vi "WriteGoodmanInfo.vi"(4 "System Pos Info":T2, 5 "error in (no error)":errorcluster, 6 "# of Entries (before)":i16, 7 "Component Names":T1, 8 "Path to FITS Header File":path) -> (0 "error out":errorcluster, 2 "# of Entries (after)":i16, 3 "Path to FITS Header File":path)   [LabVIEW 2015]
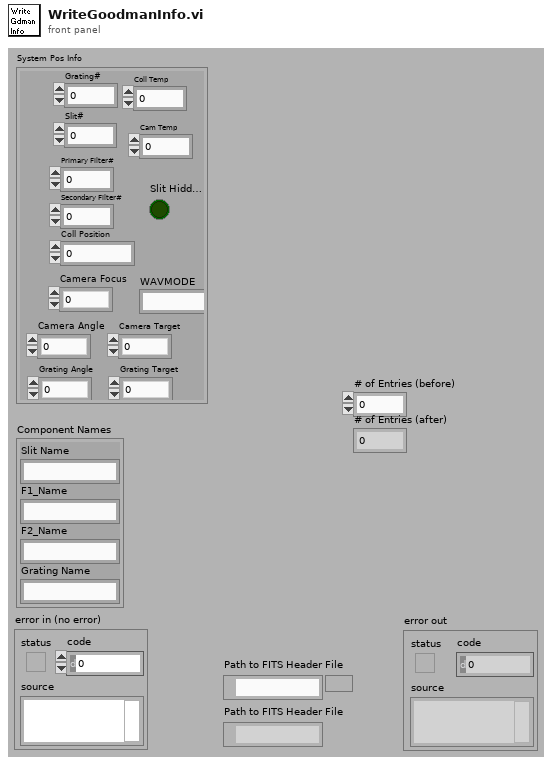
[diagram p1: front panel]
types:
  T1 = cluster{"Slit Name":string, "F1_Name":string, "F2_Name":string, "Grating Name":string}
  T2 = cluster{"Grating#":i32, "Slit#":i32, "Primary Filter#":i32, "Secondary Filter#":i32, "Coll Position":i32, "Camera Focus":i32, "Camera Angle":dbl, "Grating Angle":dbl, "Coll Temp":dbl, "Cam Temp":dbl, "Camera Target":dbl, "Grating Target":dbl, "WAVMODE":string, "Slit Hidden?":bool}
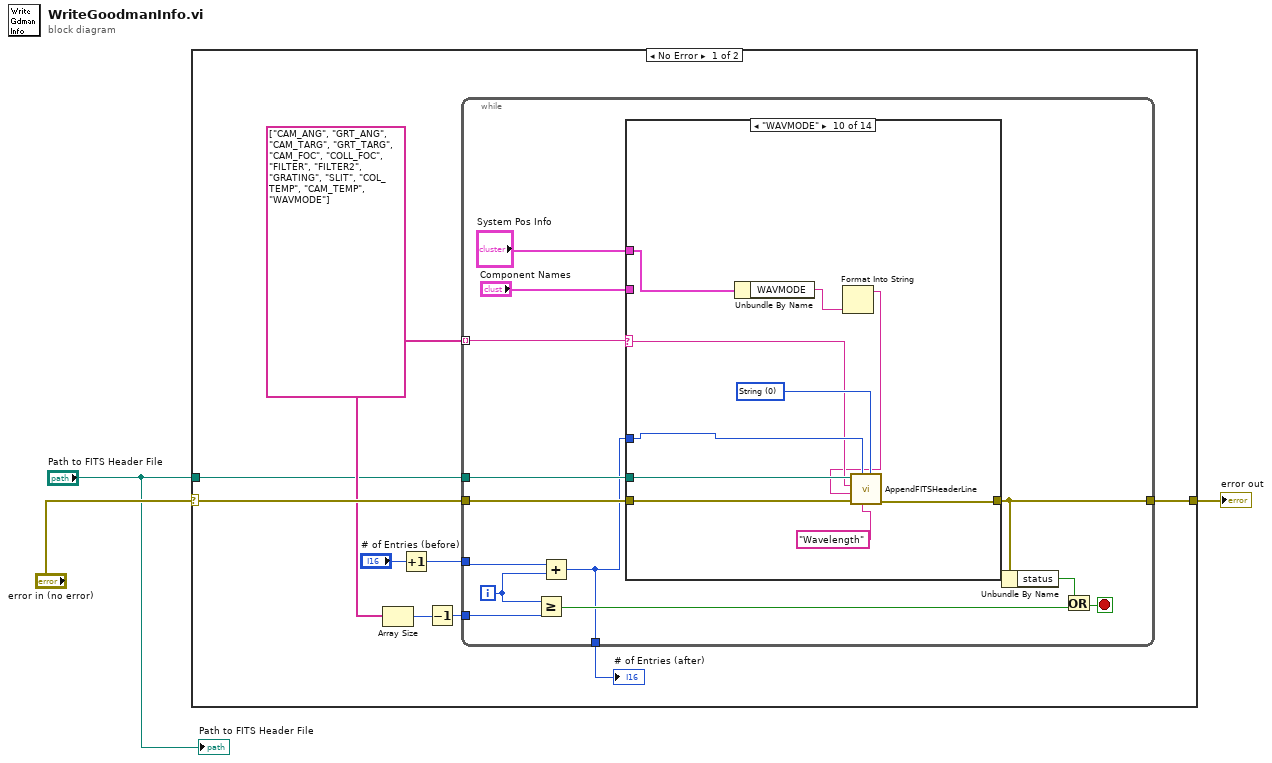
[diagram p0: block diagram]
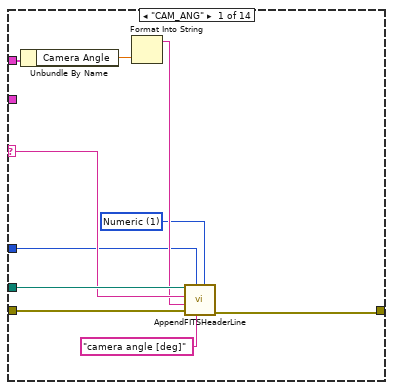
[diagram p2: hidden frame]
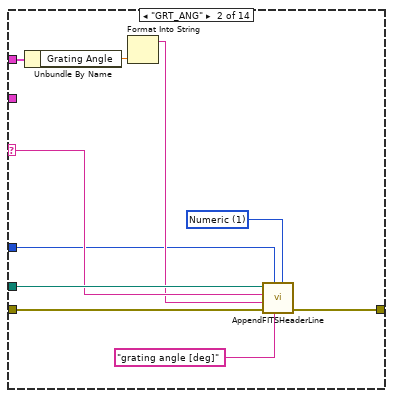
[diagram p3: hidden frame]
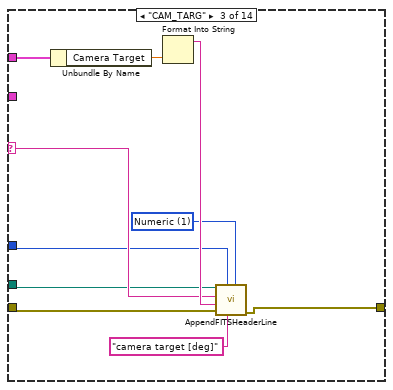
[diagram p4: hidden frame]
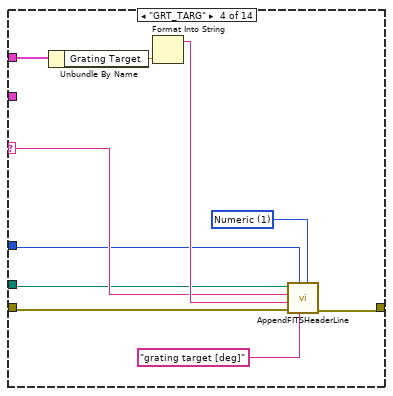
[diagram p5: hidden frame]
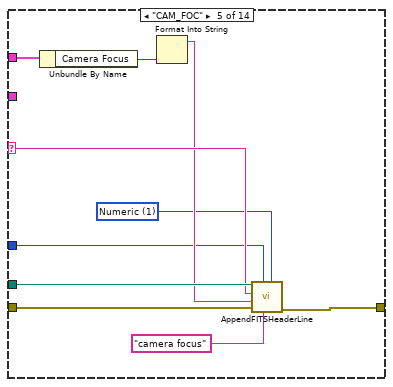
[diagram p6: hidden frame]
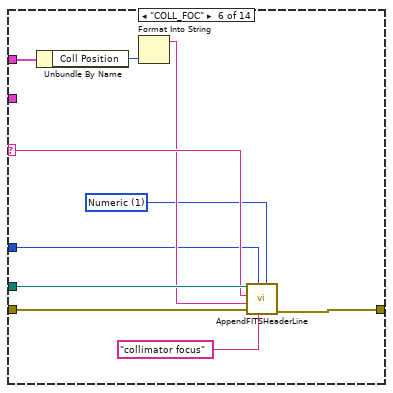
[diagram p7: hidden frame]
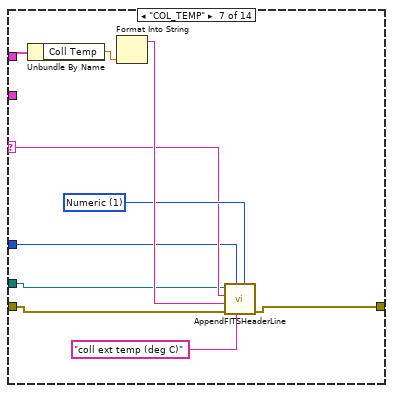
[diagram p8: hidden frame]
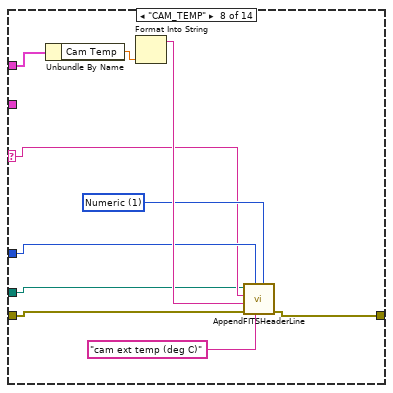
[diagram p9: hidden frame]
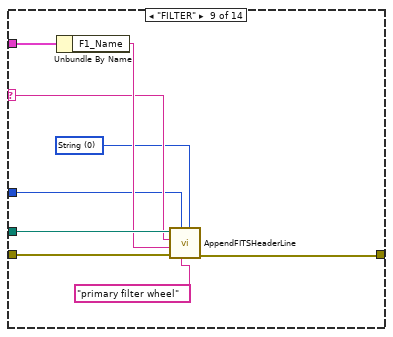
[diagram p10: hidden frame]
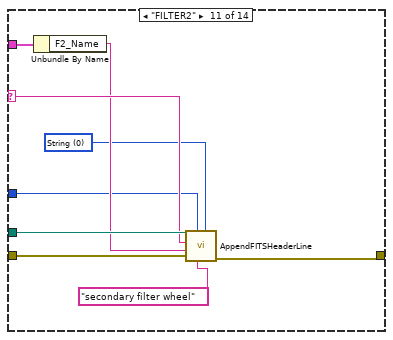
[diagram p11: hidden frame]
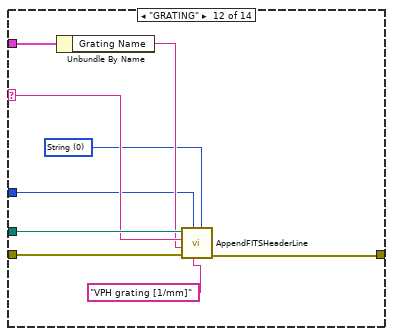
[diagram p12: hidden frame]
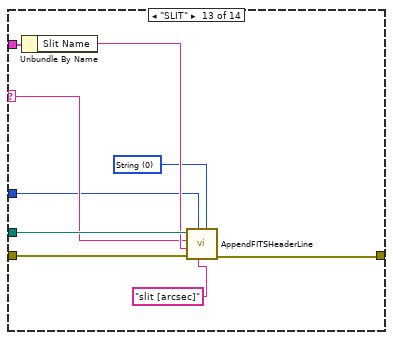
[diagram p13: hidden frame]
diagram:
  n1 = case shown="No Error" "error in (no error)" {
    selector: "error in (no error)" -> [w12 w153]
    tunnel: [w8 w153] -> w2
    tunnel: "Path to FITS Header File" -> [w7 _]
    frame No Error {
      w11 = string[] ["CAM_ANG", "GRT_ANG", "CAM_TARG", "GRT_TARG", "CAM_FOC", "COLL_FOC", "FILTER", "FILTER2", "GRATING", "SLIT", "COL_TEMP", "CAM_TEMP", "WAVMODE"]
      n2 = Array Size(array=w11) -> (size(s)=w10:i32)
      n3 = Increment(x="# of Entries (before)") -> (x+1=w5:i16)
      n4 = Decrement(x=w10) -> (x-1=w9:i32)
      n5 = while {
        tunnel: w12 -> [w25]
        tunnel: w11 -> [w23] mode=indexing
        tunnel: w9 -> [w22]
        tunnel: [w21] -> w8
        tunnel: w7 -> [w16]
        tunnel: w5 -> [w15]
        tunnel: [w13] -> w4
        i -> [w14]
        stop <- w24 stop-if-true
        n6 = Greater Or Equal?(x=w14, y=w22) -> (x >= y?=w20:bool)
        n7 = Add(x=w15, y=w14) -> (x+y=w13:i32)
        n8 = case shown="\"WAVMODE\"" w23 {
          selector: w23 -> [w31 w41 w50 w60 w70 w80 w88 w99 w109 w117 w129 w138 w146 _]
          tunnel: w25 -> [w34 w44 w47 w57 w73 w83 w92 w101 w113 w120 w132 w141 w150 w152]
          tunnel: [w33 w43 w46 w56 w72 w82 w91 w97 w111 w119 w131 w140 w149 w152] -> w21
          tunnel: "System Pos Info" -> [w35 w45 w51 w61 w75 w85 w90 w98 _ w118 _ _ _ _]
          tunnel: "Component Names" -> [_ _ _ _ _ _ _ _ w114 _ w133 w142 w151 _]
          tunnel: w16 -> [w32 w42 w48 w58 w71 w81 w86 w96 w112 w121 w130 w139 w148 _]
          tunnel: w13 -> [w27 w37 w49 w59 w67 w77 w87 w100 w108 w122 w126 w136 w145 _]
          frame "CAM_ANG" {
            w28 = u16 1 items=["String", "Numeric", "Boolean"] ("Entry Type")
            n9 = Unbundle By Name(w35) -> ("Camera Angle"=w30:dbl)
            n10 = Format Into String(w30) -> (resulting string=w29:string)  [unwired: 3 in, 1 out]
            n11 = call "AppendFITSHeaderLine.vi"("Entry Type"=w28, "Comment"="camera angle [deg]", "Entry #"=w27, "error in (no error)"=w34, "Element Value"=w29, "Element Name"=w31, "file path (dialog if empty)"=w32) -> ("error out"=w33:errorcluster)  [unwired: 3 in]
          }
          frame "GRT_ANG" {
            w38 = u16 1 items=["String", "Numeric", "Boolean"] ("Entry Type")
            n12 = Unbundle By Name(w45) -> ("Grating Angle"=w40:dbl)
            n13 = Format Into String(w40) -> (resulting string=w39:string)  [unwired: 3 in, 1 out]
            n14 = call "AppendFITSHeaderLine.vi"("Entry Type"=w38, "Comment"="grating angle [deg]", "Entry #"=w37, "error in (no error)"=w44, "Element Value"=w39, "Element Name"=w41, "file path (dialog if empty)"=w42) -> ("error out"=w43:errorcluster)  [unwired: 3 in]
          }
          frame "CAM_TARG" {
            w53 = u16 1 items=["String", "Numeric", "Boolean"] ("Entry Type")
            n15 = Unbundle By Name(w51) -> ("Camera Target"=w55:dbl)
            n16 = Format Into String(w55) -> (resulting string=w54:string)  [unwired: 3 in, 1 out]
            n17 = call "AppendFITSHeaderLine.vi"("Entry Type"=w53, "Comment"="camera target [deg]", "Entry #"=w49, "error in (no error)"=w47, "Element Value"=w54, "Element Name"=w50, "file path (dialog if empty)"=w48) -> ("error out"=w46:errorcluster)  [unwired: 3 in]
          }
          frame "GRT_TARG" {
            w63 = u16 1 items=["String", "Numeric", "Boolean"] ("Entry Type")
            n18 = Unbundle By Name(w61) -> ("Grating Target"=w65:dbl)
            n19 = Format Into String(w65) -> (resulting string=w64:string)  [unwired: 3 in, 1 out]
            n20 = call "AppendFITSHeaderLine.vi"("Entry Type"=w63, "Comment"="grating target [deg]", "Entry #"=w59, "error in (no error)"=w57, "Element Value"=w64, "Element Name"=w60, "file path (dialog if empty)"=w58) -> ("error out"=w56:errorcluster)  [unwired: 3 in]
          }
          frame "CAM_FOC" {
            w68 = u16 1 items=["String", "Numeric", "Boolean"] ("Entry Type")
            n21 = Unbundle By Name(w75) -> ("Camera Focus"=w74:i32)
            n22 = Format Into String(w74) -> (resulting string=w69:string)  [unwired: 3 in, 1 out]
            n23 = call "AppendFITSHeaderLine.vi"("Entry Type"=w68, "Comment"="camera focus", "Entry #"=w67, "error in (no error)"=w73, "Element Value"=w69, "Element Name"=w70, "file path (dialog if empty)"=w71) -> ("error out"=w72:errorcluster)  [unwired: 3 in]
          }
          frame "COLL_FOC" {
            w78 = u16 1 items=["String", "Numeric", "Boolean"] ("Entry Type")
            n24 = Unbundle By Name(w85) -> ("Coll Position"=w84:i32)
            n25 = Format Into String(w84) -> (resulting string=w79:string)  [unwired: 3 in, 1 out]
            n26 = call "AppendFITSHeaderLine.vi"("Entry Type"=w78, "Comment"="collimator focus", "Entry #"=w77, "error in (no error)"=w83, "Element Value"=w79, "Element Name"=w80, "file path (dialog if empty)"=w81) -> ("error out"=w82:errorcluster)  [unwired: 3 in]
          }
          frame "COL_TEMP" {
            w94 = u16 1 items=["String", "Numeric", "Boolean"] ("Entry Type")
            n27 = Unbundle By Name(w90) -> ("Coll Temp"=w89:dbl)
            n28 = Format Into String(w89) -> (resulting string=w95:string)  [unwired: 3 in, 1 out]
            n29 = call "AppendFITSHeaderLine.vi"("Entry Type"=w94, "Comment"="coll ext temp (deg C)", "Entry #"=w87, "error in (no error)"=w92, "Element Value"=w95, "Element Name"=w88, "file path (dialog if empty)"=w86) -> ("error out"=w91:errorcluster)  [unwired: 3 in]
          }
          frame "CAM_TEMP" {
            w104 = u16 1 items=["String", "Numeric", "Boolean"] ("Entry Type")
            n30 = Unbundle By Name(w98) -> ("Cam Temp"=w102:dbl)
            n31 = Format Into String(w102) -> (resulting string=w105:string)  [unwired: 3 in, 1 out]
            n32 = call "AppendFITSHeaderLine.vi"("Entry Type"=w104, "Comment"="cam ext temp (deg C)", "Entry #"=w100, "error in (no error)"=w101, "Element Value"=w105, "Element Name"=w99, "file path (dialog if empty)"=w96) -> ("error out"=w97:errorcluster)  [unwired: 3 in]
          }
          frame "FILTER" {
            w107 = u16 0 items=["String", "Numeric", "Boolean"] ("Entry Type")
            n33 = Unbundle By Name(w114) -> ("F1_Name"=w110:string)
            n34 = call "AppendFITSHeaderLine.vi"("Entry Type"=w107, "Comment"="primary filter wheel", "Entry #"=w108, "error in (no error)"=w113, "Element Value"=w110, "Element Name"=w109, "file path (dialog if empty)"=w112) -> ("error out"=w111:errorcluster)  [unwired: 3 in]
          }
          frame "WAVMODE" {
            w124 = u16 0 items=["String", "Numeric", "Boolean"] ("Entry Type")
            n35 = Unbundle By Name(w118) -> ("WAVMODE"=w116:string)
            n36 = Format Into String(w116) -> (resulting string=w115:string)  [unwired: 3 in, 1 out]
            n37 = call "AppendFITSHeaderLine.vi"("Entry Type"=w124, "Comment"="Wavelength", "Entry #"=w122, "error in (no error)"=w120, "Element Value"=w115, "Element Name"=w117, "file path (dialog if empty)"=w121) -> ("error out"=w119:errorcluster)  [unwired: 3 in]
          }
          frame "FILTER2" {
            w127 = u16 0 items=["String", "Numeric", "Boolean"] ("Entry Type")
            n38 = Unbundle By Name(w133) -> ("F2_Name"=w128:string)
            n39 = call "AppendFITSHeaderLine.vi"("Entry Type"=w127, "Comment"="secondary filter wheel", "Entry #"=w126, "error in (no error)"=w132, "Element Value"=w128, "Element Name"=w129, "file path (dialog if empty)"=w130) -> ("error out"=w131:errorcluster)  [unwired: 3 in]
          }
          frame "GRATING" {
            w135 = u16 0 items=["String", "Numeric", "Boolean"] ("Entry Type")
            n40 = Unbundle By Name(w142) -> ("Grating Name"=w137:string)
            n41 = call "AppendFITSHeaderLine.vi"("Entry Type"=w135, "Comment"="VPH grating [1/mm]", "Entry #"=w136, "error in (no error)"=w141, "Element Value"=w137, "Element Name"=w138, "file path (dialog if empty)"=w139) -> ("error out"=w140:errorcluster)  [unwired: 3 in]
          }
          frame "SLIT" {
            w144 = u16 0 items=["String", "Numeric", "Boolean"] ("Entry Type")
            n42 = Unbundle By Name(w151) -> ("Slit Name"=w147:string)
            n43 = call "AppendFITSHeaderLine.vi"("Entry Type"=w144, "Comment"="slit [arcsec]", "Entry #"=w145, "error in (no error)"=w150, "Element Value"=w147, "Element Name"=w146, "file path (dialog if empty)"=w148) -> ("error out"=w149:errorcluster)  [unwired: 3 in]
          }
          frame "", Default {
          }
        }
        n44 = Unbundle By Name(w21) -> ("status"=w19:bool)
        n45 = Or(x=w19, y=w20) -> (x .or. y?=w24:bool)
      }
      "# of Entries (after)" <- w4
    }
    frame Error {
    }
  }
  "error out" <- w2
  "Path to FITS Header File" <- "Path to FITS Header File"
